vi "关闭设备.vi"(10 "设备句柄":i32 min=0 max=50) -> ()   [LabVIEW 2016]
uses:
  dll/em9636.dll
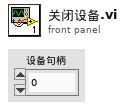
[diagram p1: front panel]
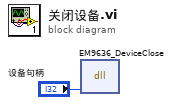
[diagram p0: block diagram]
diagram:
  n1 = dll-call lib="PTH2kabs CUsers\nAdministratorDesktopEM9636*EM9636系列_demo_labview(调用DLL方式)dll\nem9636.dll" fn="EM9636_DeviceClose"("设备句柄"="设备句柄") -> ()  [unwired: 5 in, 2 out]
